vi "Buttons Latching Write.vi"(4 "error in (no error)":errorcluster, 5 "Value":bool[](array[boolean]), 6 "Container State":T3, 7 "Display State In":T1={"Buttons Displayed"=0, "Button States"=[], "Button Size"=0, "Button Style"=enum."Classic", "Active Button"=0, "Force Regen?"=FALSE, "Tip String Ref"=refnum}) -> (0 "error out":errorcluster, 3 "Display State Out":T1={"Buttons Displayed"=0, "Button States"=[], "Button Size"=0, "Button Style"=enum."Classic", "Active Button"=0, "Force Regen?"=FALSE, "Tip String Ref"=refnum})   [LabVIEW 2012, in "Toolbar.xctl"]
doc: "Set which of the toolbar buttons are latching and which are transitory. (T=Latching, F=Transitory)"
uses:
  Toolbar.xctl
  <vilib>/_xctls/Container State.ctl
  Toolbar State.ctl
  Button_Class/Button.lvclass
  Button_Class/Type Defs/Button Style.ctl
  Button_Class/Type Defs/Button Type.ctl
  <vilib>/_xctls/XControlSupport.lvlib
panel:
  # "Replace the Value Control below with a Control of desired type.\nDo not remove this Control or the others from the connector pane.\nDo not change the connector pane pattern.\nThe Value control should always be the third terminal from top on the input side in the connector pane."
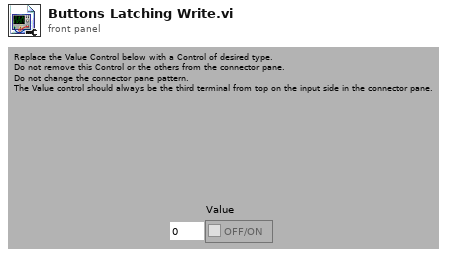
[diagram p1: front panel]
types:
  T1 = typedef "Toolbar.xctl/Toolbar State.ctl" = cluster{"Buttons Displayed":i32, "Button States":refnum<class "Button.lvclass">[], "Button Size":i32, "Button Style":T2, "Active Button":i32, "Force Regen?":bool, "Tip String Ref":refnum<vi>}
  T2 = typedef "Button.lvclass/Button Style.ctl" = enum16{"System", "Modern", "Classic", "Rounded", "Silver", "Ni Theme", "Metallic"}
  T3 = typedef "XControlSupport.lvlib/Container State.ctl" = cluster{"Indicator?":bool, "Run Mode?":bool, " Refnum":refnum<vi>}
  T4 = typedef "Button.lvclass/Button Type.ctl" = enum16{"Transitory", "Latching"}
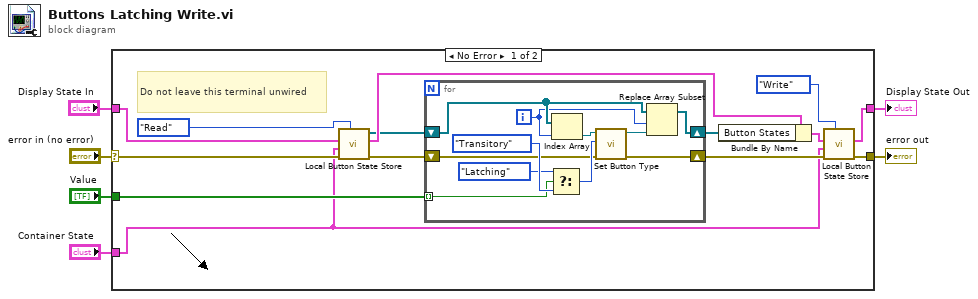
[diagram p0: block diagram]
diagram:
  n1 = case shown="No Error" "error in (no error)" {
    selector: "error in (no error)" -> [w19 w33]
    tunnel: "Value" -> [w20 _]
    tunnel: [w15 w33] -> w4
    tunnel: [w11 w32] -> w3
    tunnel: "Container State" -> [w10 _]
    tunnel: "Display State In" -> [w9 w32]
    frame No Error {
      # "Do not leave this terminal unwired"
      n2 = call "Local Button State Store.vi"("Operation"=enum16{"Read", "Write"}."Read", "error in (no error)"=w19, "Container State"=w10, "Display State In"=w9) -> ("error out"=w18:errorcluster, "Display State Out"=w8:T1, "Button States"=w7:refnum<class "Button.lvclass">[])  [unwired: 5 out]
      n3 = for {
        shift-right: [w30] -> w14
        shift-left: w7 -> [w31]
        tunnel: w20 -> [w26] mode=indexing
        shift-right: [w21] -> w16
        shift-left: w18 -> [w22]
        i -> [w29]
        n4 = Select(t=Button_Type."Latching" ("Type"), s=w26, f=Button_Type."Transitory" ("Type")) -> (s? t:f=w23:T4)
        n5 = Index Array(array=w31, index=w29) -> (element=w25:refnum<class "Button.lvclass">)
        n6 = call-dynamic "Set Button Type.vi"("error in (no error)"=w22, "Type"=w23, "Button in"=w25) -> ("error out"=w21:errorcluster, "Button out"=w24:refnum<class "Button.lvclass">)  [unwired: 7 out]
        n7 = Replace Array Subset(array=w31, new element=w24, index=w29) -> (w30:refnum<class "Button.lvclass">[])
      }
      n8 = Bundle By Name(cluster=w8, "Button States"=w14) -> (w12:T1)
      n9 = call "Local Button State Store.vi"("Operation"=enum16{"Read", "Write"}."Write", "error in (no error)"=w16, "Container State"=w10, "Display State In"=w12) -> ("error out"=w15:errorcluster, "Display State Out"=w11:T1)  [unwired: 1 in, 5 out]
    }
    frame Error {
    }
  }
  "error out" <- w4
  "Display State Out" <- w3
